vi "Read Array Key (Boolean).vi"(7 "Section Name":string, 8 "error in (no error)":errorcluster, 9 "Default":bool, 10 "Key Name":string, 11 "Config in":refnum<class "LabVIEW-Config.lvclass">) -> (0 "error out":errorcluster, 1 "Value":bool[](array[boolean]), 3 "Config out":refnum<class "LabVIEW-Config.lvclass">)   [LabVIEW 2017, in "LabVIEW-Config.lvlib" / "LabVIEW-Config.lvclass"]
uses:
  LabVIEW-Config.lvclass
panel:
  out "Key Found?":bool
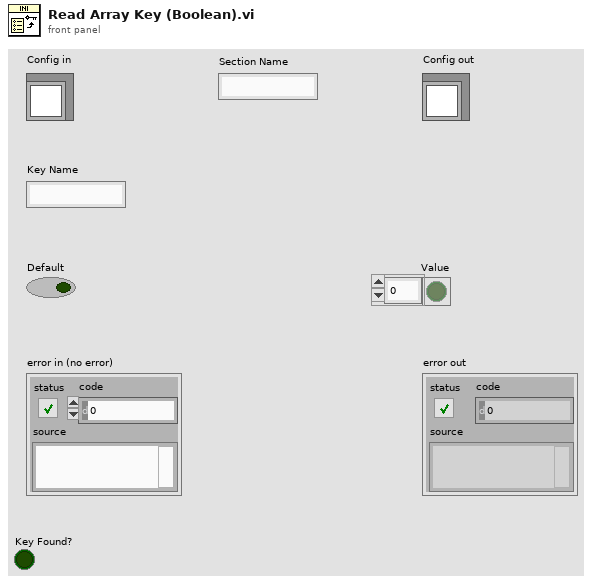
[diagram p1: front panel]
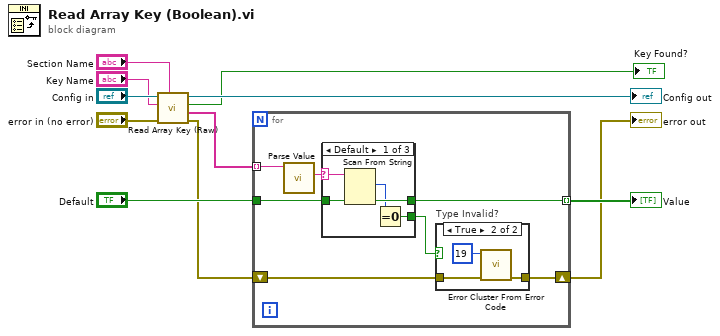
[diagram p0: block diagram]
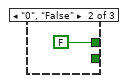
[diagram p2: hidden frame]
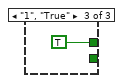
[diagram p3: hidden frame]
diagram:
  n1 = call "Read Array Key (Raw).vi"("Section Name"="Section Name", "error in (no error)"="error in (no error)", "Key Name"="Key Name", "Config in"="Config in") -> ("error out"=w2:errorcluster, "Content"=w6:string[], "Key Found?"=→"Key Found?":bool, "Config out"=→"Config out":refnum<class "LabVIEW-Config.lvclass">)  [unwired: 4 in]
  n2 = for {
    tunnel: w6 -> [w18] mode=indexing
    shift-right: [w15] -> w3
    shift-left: w2 -> [w14]
    tunnel: "Default" -> [w16]
    tunnel: [w17] -> w5 mode=indexing
    n3 = call "Parse Value.vi"("Value"=w18) -> ("Value (Comment Removed)"=w13:string)  [unwired: 9 in, 1 out]
    n4 = case shown="Default" w13 {
      selector: w13 -> [w23 _ _]
      tunnel: [w22 FALSE TRUE] -> w17
      tunnel: [w20 _ _] -> w12
      tunnel: w16 -> [w19 _ _]
      frame Default {
        n5 = Scan From String(input string=w23, default 1=w19) -> (offset past scan=w21:u32, output 1=w22:bool)  [unwired: 3 in, 2 out]
        n6 = Equal To 0?(x=w21) -> (x = 0?=w20:bool)
      }
      frame "0", "False" {
      }
      frame "1", "True" {
      }
    }
    n7 = case "Type Invalid?" shown="True" w12 {
      tunnel: w14 -> [w26 w28]
      tunnel: [w26 w27] -> w15
      frame False {
      }
      frame True {
        n8 = call <vilib>:"Error Cluster From Error Code.vi"("error in (no error)"=w28, "error code (0)"=19 ("Type invalid")) -> ("error out"=w27:errorcluster)  [unwired: 7 in]
      }
    }
  }
  "error out" <- w3
  "Value" <- w5
